vi "Configure Offset And Limits List (Multi-Carrier Power).vi"(0 "VISA resource name":refnum<visa-resource-name>, 1 "Upper Offset Limit":dbl[](array[numeric])=[0.0, 0.0, 0.0] format="%#.6g", 2 "Lower Offset Limit":dbl[](array[numeric])=[0.0, 0.0, 0.0] format="%#.6g", 5 "Frequency Offsets (5 MHz, 10 MHz, 15 MHz)":dbl[](array[numeric])=[5000000.0, 10000000.0, 15000000.0] format="%#.6g", 7 "Offset Integration Bandwidth (3.84 MHz, 3.84 MHz, 3.84 MHz)":dbl[](array[numeric])=[3840000.0, 3840000.0, 3840000.0] format="%#.6g", 11 "error in (no error)":errorcluster) -> (4 "VISA resource name out":refnum<visa-resource-name>, 15 "error out":errorcluster)   [LabVIEW 2014, in "Agilent ESA PSA Series.lvlib"]
doc: "Sets up the limit and frequency of multi carrier power measurement."
uses:
  Agilent ESA PSA Series.lvlib
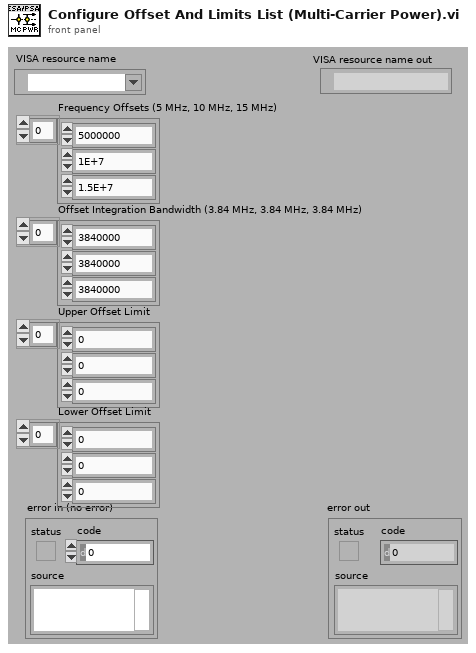
[diagram p1: front panel]
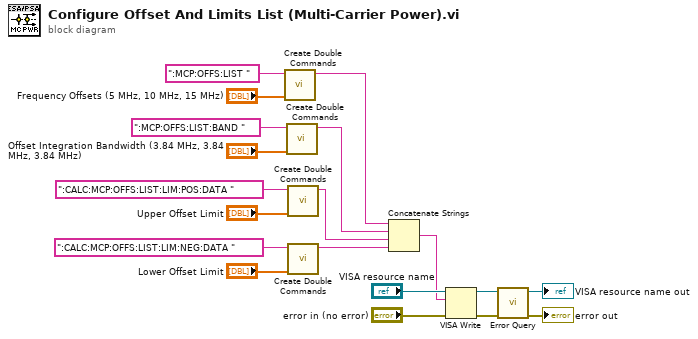
[diagram p0: block diagram]
diagram:
  n1 = call "Create Double Commands.vi"("Double Values"="Frequency Offsets (5 MHz, 10 MHz, 15 MHz)", "Commands"=":MCP:OFFS:LIST ") -> ("Result"=w1:string)  [unwired: 9 in]
  n2 = call "Create Double Commands.vi"("Double Values"="Offset Integration Bandwidth (3.84 MHz, 3.84 MHz, 3.84 MHz)", "Commands"=":MCP:OFFS:LIST:BAND ") -> ("Result"=w2:string)  [unwired: 9 in]
  n3 = call "Create Double Commands.vi"("Double Values"="Upper Offset Limit", "Commands"=":CALC:MCP:OFFS:LIST:LIM:POS:DATA ") -> ("Result"=w3:string)  [unwired: 9 in]
  n4 = call "Create Double Commands.vi"("Double Values"="Lower Offset Limit", "Commands"=":CALC:MCP:OFFS:LIST:LIM:NEG:DATA ") -> ("Result"=w4:string)  [unwired: 9 in]
  n5 = Concatenate Strings(w1, w2, w3, w4) -> (w13:string)
  n6 = VISA Write(VISA resource name="VISA resource name", write buffer=w13, error in (no error)="error in (no error)") -> (VISA resource name out=w19:refnum<visa-resource-name>, error out=w18:errorcluster)  [unwired: 1 out]
  n7 = call "Error Query.vi"("error in (no error)"=w18, "VISA resource name"=w19) -> ("error out"=→"error out":errorcluster, "VISA resource name out"=→"VISA resource name out":refnum<visa-resource-name>)  [unwired: 6 in, 2 out]
